vi "Error.vi"(8 "error in":errorcluster, 11 "Ignore Errors (Runtime)":i32[](array[numeric])) -> (0 "error out":errorcluster)   [LabVIEW 2015]
uses:
  Message Queue/Message Queue.lvlib
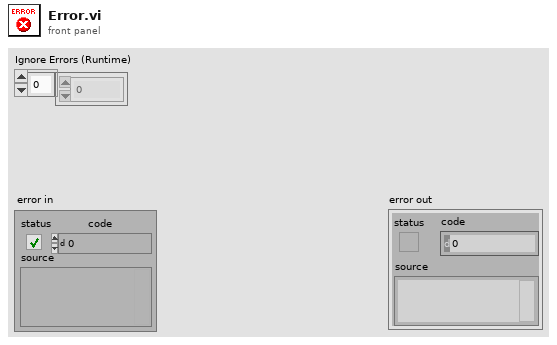
[diagram p1: front panel]
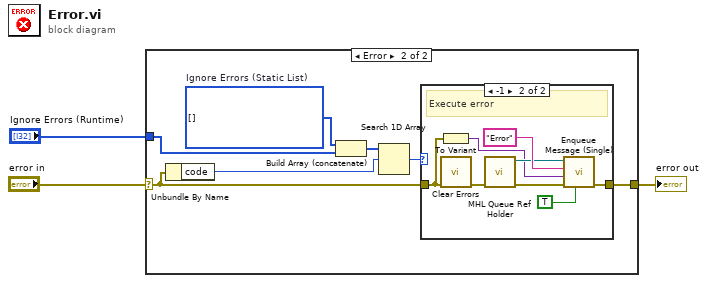
[diagram p0: block diagram]
diagram:
  n1 = case shown="Error" "error in" {
    selector: "error in" -> [w4 w6]
    tunnel: [w4 w11] -> w3
    tunnel: "Ignore Errors (Runtime)" -> [_ w7]
    frame No Error {
    }
    frame Error {
      w8 = i32[] []  # Ignore Errors (Static List)
      n2 = Unbundle By Name(w6) -> ("code"=w10:i32)
      n3 = Build Array (concatenate)(w8, w7) -> (w9:i32[])
      n4 = Search 1D Array(1D array=w9, element=w10) -> (index of element=w5:i32)  [unwired: 1 in]
      n5 = case shown="-1" w5 {
        tunnel: w6 -> [w12 w15]
        tunnel: [w12 w13] -> w11
        frame Default {
          # "Ignore error"
        }
        frame -1 {
          # "Execute error"
          n6 = To Variant(anything=w15) -> (Variant=w17:variant)
          n7 = call <vilib>:"Clear Errors.vi"("error in (no error)"=w15) -> ("error out"=w14:errorcluster)  [unwired: 5 in, 1 out]
          n8 = call "MHL Queue Ref Holder.vi"("error in"=w14) -> ("error out"=w18:errorcluster, "Input Message Queue"=w19:refnum<queue>)  [unwired: 9 in]
          n9 = call "Enqueue Message (Single).vi"("Priority Message? (F)"=TRUE, "error in (no error)"=w18, "Message Data"=w17, "Message"="Error", "Message Queue"=w19) -> ("error out"=w13:errorcluster)  [unwired: 5 in, 1 out]
        }
      }
    }
  }
  "error out" <- w3
